vi "Get Buffer Status.vi"(8 "error in":errorcluster, 11 "Buffer in":refnum<data-value>) -> (0 "error out":errorcluster, 1 "bufSize":i32, 2 "nbElements":i32, 3 "Buffer":refnum<data-value>, 4 "full":bool)   [LabVIEW 2013, in "VariantBuffer.lvclass"]
doc: "This VI returns data from the ring buffer starting from the oldest data and ending with the newest.\n\nThe data is duplicated at the output so this VI allocates new place in the memory for the output."
uses:
  VariantBuffer.lvclass
  VariantBuffer.lvclass/VariantBuffer.ctl
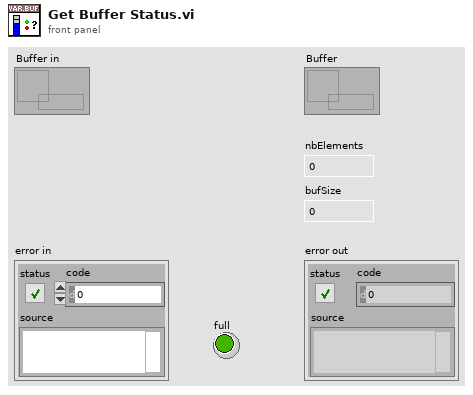
[diagram p1: front panel]
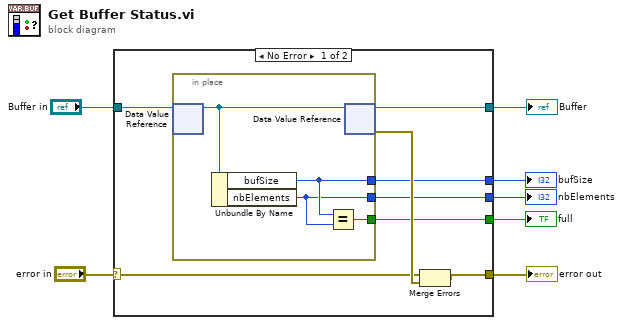
[diagram p0: block diagram]
diagram:
  n1 = case shown="No Error" "error in" {
    selector: "error in" -> [w10 w20]
    tunnel: "Buffer in" -> [w15 w21]
    tunnel: [w14 w21] -> w6
    tunnel: [w12 w20] -> w3
    tunnel: [w11 _] -> w5
    tunnel: [w9 _] -> w2
    tunnel: [w8 _] -> w1
    frame No Error {
      n2 = in-place {
        in-place-border: [w17] -> w11
        in-place-border: [w18] -> w9
        in-place-border: [w16] -> w8
        n3 = in-place-dvr #1(w15) -> (w19:refnum<class "VariantBuffer.lvclass">)  [unwired: 1 out]
        n4 = Unbundle By Name(w19) -> ("bufSize"=w18:i32, "nbElements"=w17:i32)
        n5 = Equal?(x=w18, y=w17) -> (x = y?=w16:bool)
        n6 = in-place-dvr #1(w19) -> (w14:refnum<data-value>, w13:errorcluster)
      }
      n7 = Merge Errors(w10, w13) -> (w12:errorcluster)
    }
    frame Error {
    }
  }
  "error out" <- w3
  "Buffer" <- w6
  "nbElements" <- w5
  "bufSize" <- w2
  "full" <- w1
